vi "asyncAcq_occurenceRef_timeStamp.vi"(0 "reference":refnum<class "OSA300.lvclass">, 5 "error in (no error)":errorcluster) -> (14 "duplicate reference":refnum<class "OSA300.lvclass">, 15 "new spectrum":bool, 16 "new interferogram":bool, 18 "error":u32, 19 "error out":errorcluster)   [LabVIEW 2010, in "OSA300.lvclass"]
doc: "Reads the contents of a <B>Thorlabs_OSA_64</B> object.\n\n[GOOP 1.0]"
uses:
  OSA300.lvclass
  OSA.lvclass
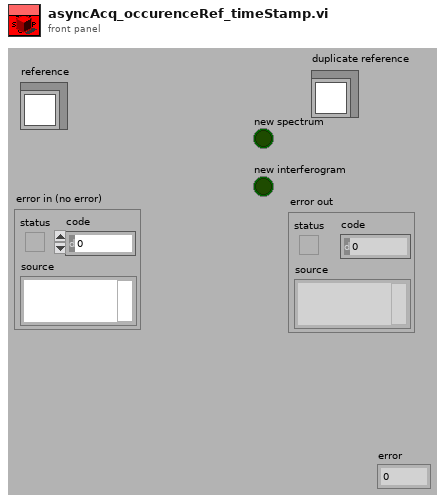
[diagram p1: front panel]
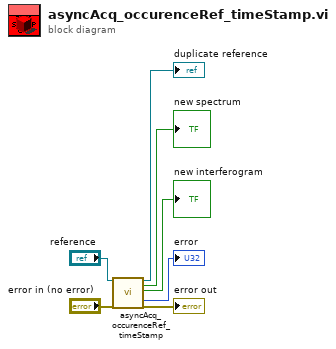
[diagram p0: block diagram]
diagram:
  n1 = call-parent "asyncAcq_occurenceRef_timeStamp.vi"("reference"="reference", "error in (no error)"="error in (no error)") -> ("duplicate reference"=→"duplicate reference":refnum<class "OSA300.lvclass">, "new spectrum"=→"new spectrum":bool, "new interferogram"=→"new interferogram":bool, "error"=→"error":u32, "error out"=→"error out":errorcluster)  [unwired: 13 in]
